vi "BRig_dataLC_ENL_PostR_Prob_l1.vi"() -> (2 "output_ENL_PostR_Prob":i32)   [LabVIEW 2014]
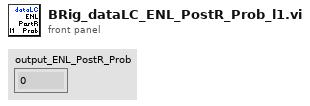
[diagram p1: front panel]
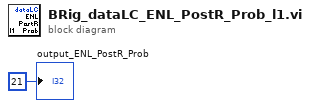
[diagram p0: block diagram]
diagram:
  "output_ENL_PostR_Prob" <- 21 ("output_iBlock")
